vi "4-6.1.vi"(1 "数值 2":dbl, 2 "数值":dbl) -> (0 "数值 3":dbl)   [LabVIEW 2017]
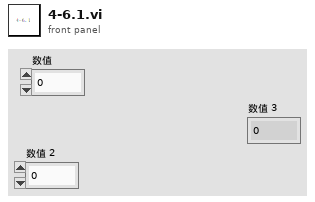
[diagram p1: front panel]
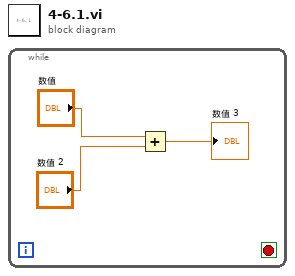
[diagram p0: block diagram]
diagram:
  n1 = while {
    stop <- _ stop-if-true
    n2 = Add(x="数值", y="数值 2") -> (x+y=→"数值 3":dbl)
  }
